vi "0_PlanVirtualStave.vi"(7 "Stave Locking Points [mm]":dbl[][](array[numeric])=[[0.0, 0.0, 0.0], [280.05, 0.0, 0.0], [574.05, 0.0, 0.0], [868.05, 0.0, 0.0], [1162.05, 0.0, 0.0]], 8 "Working height [mm]":dbl, 9 "N Modules":i32=13, 10 "Module fiducial marker":T3(ring), 11 "Tape Type":enum16{"Stereo", "Axial"}(ring)=enum."Axial") -> (0 "Module fiducials in the Stave's basis":T1(graph)=[{"Generated List of Module Coordinates"=[0.0, 280.05, 574.05, 868.05, 1162.05], "Generated List of Module Coordinates"=[0.0, 0.0, 0.0, 0.0, 0.0]}, {"Generated List of Module Coordinates"=[-7.689999999999998, 87.79, 87.79, -7.689999999999998, 90.31, 185.79000000000002, 185.79000000000002, 90.31, 188.31, 283.79, 283.79, 188.31, 286.31, 381.79, 381.79, 286.31, 384.31, 479.79, 479.79, 384.31, 482.30999999999995, 577.79, 577.79, 482.30999999999995, 580.31, 675.79, 675.79, 580.31, 678.31, 773.79, 773.79, 678.31, 776.31, 871.79, 871.79, 776.31, 874.31, 969.79, 969.79, 874.31, 972.31, 1067.79, 1067.79, 972.31, 1070.31, 1165.79, 1165.79, 1070.31, 1168.31, 1263.79, 1263.79, 1168.31], "Generated List of Module Coordinates"=[-113.212, -113.212, -16.13199999999999, -16.13199999999999, -113.212, -113.212, -16.13199999999999, -16.13199999999999, -113.212, -113.212, -16.13199999999999, -16.13199999999999, -113.212, -113.212, -16.13199999999999, -16.13199999999999, -113.212, -113.212, -16.13199999999999, -16.13199999999999, -113.212, -113.212, -16.13199999999999, -16.13199999999999, -113.212, -113.212, -16.13199999999999, -16.13199999999999, -113.212, -113.212, -16.13199999999999, -16.13199999999999, -113.212, -113.212, -16.13199999999999, -16.13199999999999, -113.212, -113.212, -16.13199999999999, -16.13199999999999, -113.212, -113.212, -16.13199999999999, -16.13199999999999, -113.212, -113.212, -16.13199999999999, -16.13199999999999, -113.212, -113.212, -16.13199999999999, -16.13199999999999]}, {"Generated List of Module Coordinates"=[40.050000000000004, 138.05, 236.05, 334.05, 432.05, 530.05, 628.05, 726.05, 824.05, 922.05, 1020.05, 1118.05, 1216.05], "Generated List of Module Coordinates"=[-64.672, -64.672, -64.672, -64.672, -64.672, -64.672, -64.672, -64.672, -64.672, -64.672, -64.672, -64.672, -64.672]}], 3 "Stave Basis: Coordinates of Fiducials on Modules":dbl[][](array[numeric])=[[-7.689999999999998, -113.212, 0.0], [87.79, -113.212, 0.0], [87.79, -16.13199999999999, 0.0], [-7.689999999999998, -16.13199999999999, 0.0], [90.31, -113.212, 0.0], [185.79000000000002, -113.212, 0.0], [185.79000000000002, -16.13199999999999, 0.0], [90.31, -16.13199999999999, 0.0], [188.31, -113.212, 0.0], [283.79, -113.212, 0.0], [283.79, -16.13199999999999, 0.0], [188.31, -16.13199999999999, 0.0], [286.31, -113.212, 0.0], [381.79, -113.212, 0.0], [381.79, -16.13199999999999, 0.0], [286.31, -16.13199999999999, 0.0], [384.31, -113.212, 0.0], [479.79, -113.212, 0.0], [479.79, -16.13199999999999, 0.0], [384.31, -16.13199999999999, 0.0], [482.30999999999995, -113.212, 0.0], [577.79, -113.212, 0.0], [577.79, -16.13199999999999, 0.0], [482.30999999999995, -16.13199999999999, 0.0], [580.31, -113.212, 0.0], [675.79, -113.212, 0.0], [675.79, -16.13199999999999, 0.0], [580.31, -16.13199999999999, 0.0], [678.31, -113.212, 0.0], [773.79, -113.212, 0.0], [773.79, -16.13199999999999, 0.0], [678.31, -16.13199999999999, 0.0], [776.31, -113.212, 0.0], [871.79, -113.212, 0.0], [871.79, -16.13199999999999, 0.0], [776.31, -16.13199999999999, 0.0], [874.31, -113.212, 0.0], [969.79, -113.212, 0.0], [969.79, -16.13199999999999, 0.0], [874.31, -16.13199999999999, 0.0], [972.31, -113.212, 0.0], [1067.79, -113.212, 0.0], [1067.79, -16.13199999999999, 0.0], [972.31, -16.13199999999999, 0.0], [1070.31, -113.212, 0.0], [1165.79, -113.212, 0.0], [1165.79, -16.13199999999999, 0.0], [1070.31, -16.13199999999999, 0.0], [1168.31, -113.212, 0.0], [1263.79, -113.212, 0.0], [1263.79, -16.13199999999999, 0.0], [1168.31, -16.13199999999999, 0.0]])   [LabVIEW 2016]
panel:
  in  "Sensor Pattern":enum16{"ATLAS07", "ATLAS12", "ATLAS17"}(ring)=enum."ATLAS12"
  in  "Stereo Angle [mrad]":dbl=40.0 format="%#_13g"
  in  "Module centre [mm]":T2
  in  "Module width [mm]":dbl=97.54
  in  "Module pitch [mm]":dbl=98.0
  # "Provided by Camera Calibration:"
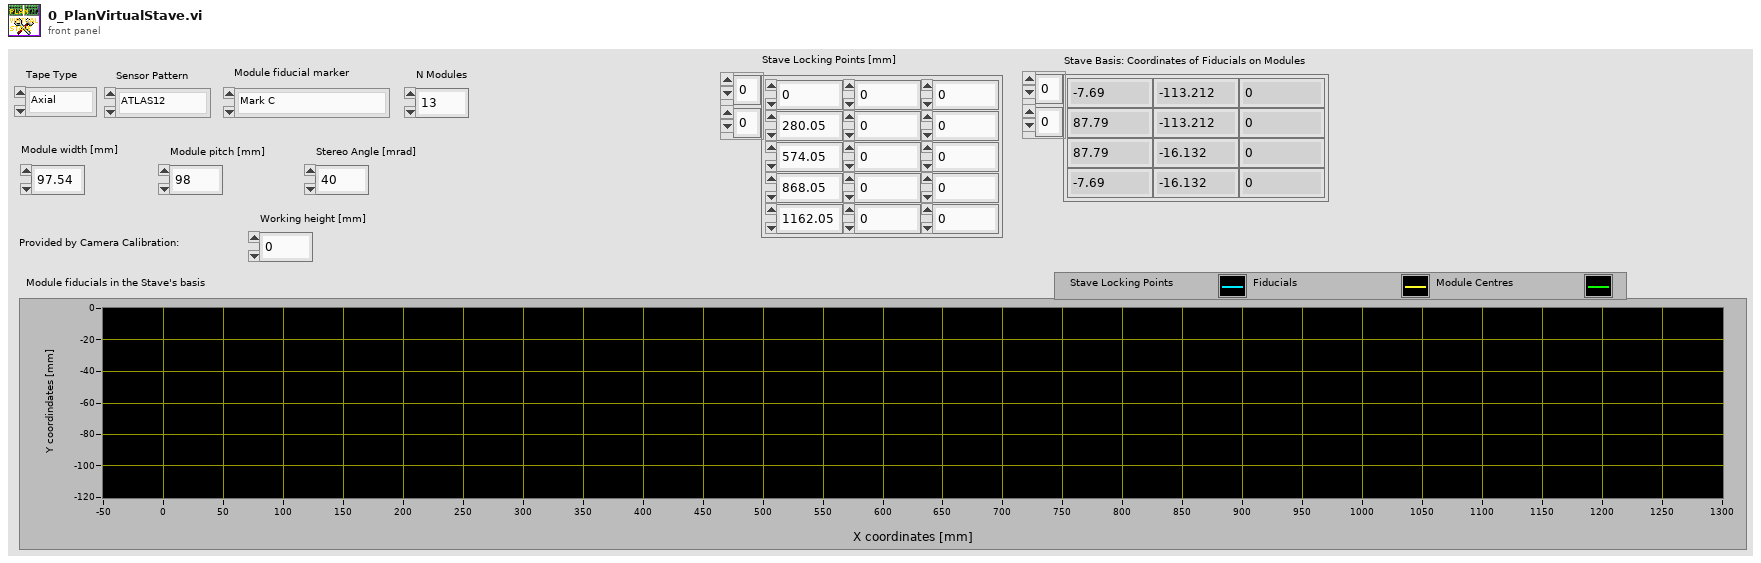
[diagram p1: front panel]
types:
  T1 = cluster{"Generated List of Module Coordinates":dbl[], "Generated List of Module Coordinates":dbl[]}[]
  T2 = cluster{"X [mm]":dbl, "Y [mm]":dbl, "Z [mm]":dbl}
  T3 = enum16{"Mark C", "Mark B", "Strip Corner", "[None]"}
  T4 = cluster{"Stave Locking Points [mm]":dbl[], "Stave Locking Points [mm]":dbl[]}
  T5 = cluster{"Generated List of Module Coordinates":dbl[], "Generated List of Module Coordinates":dbl[]}
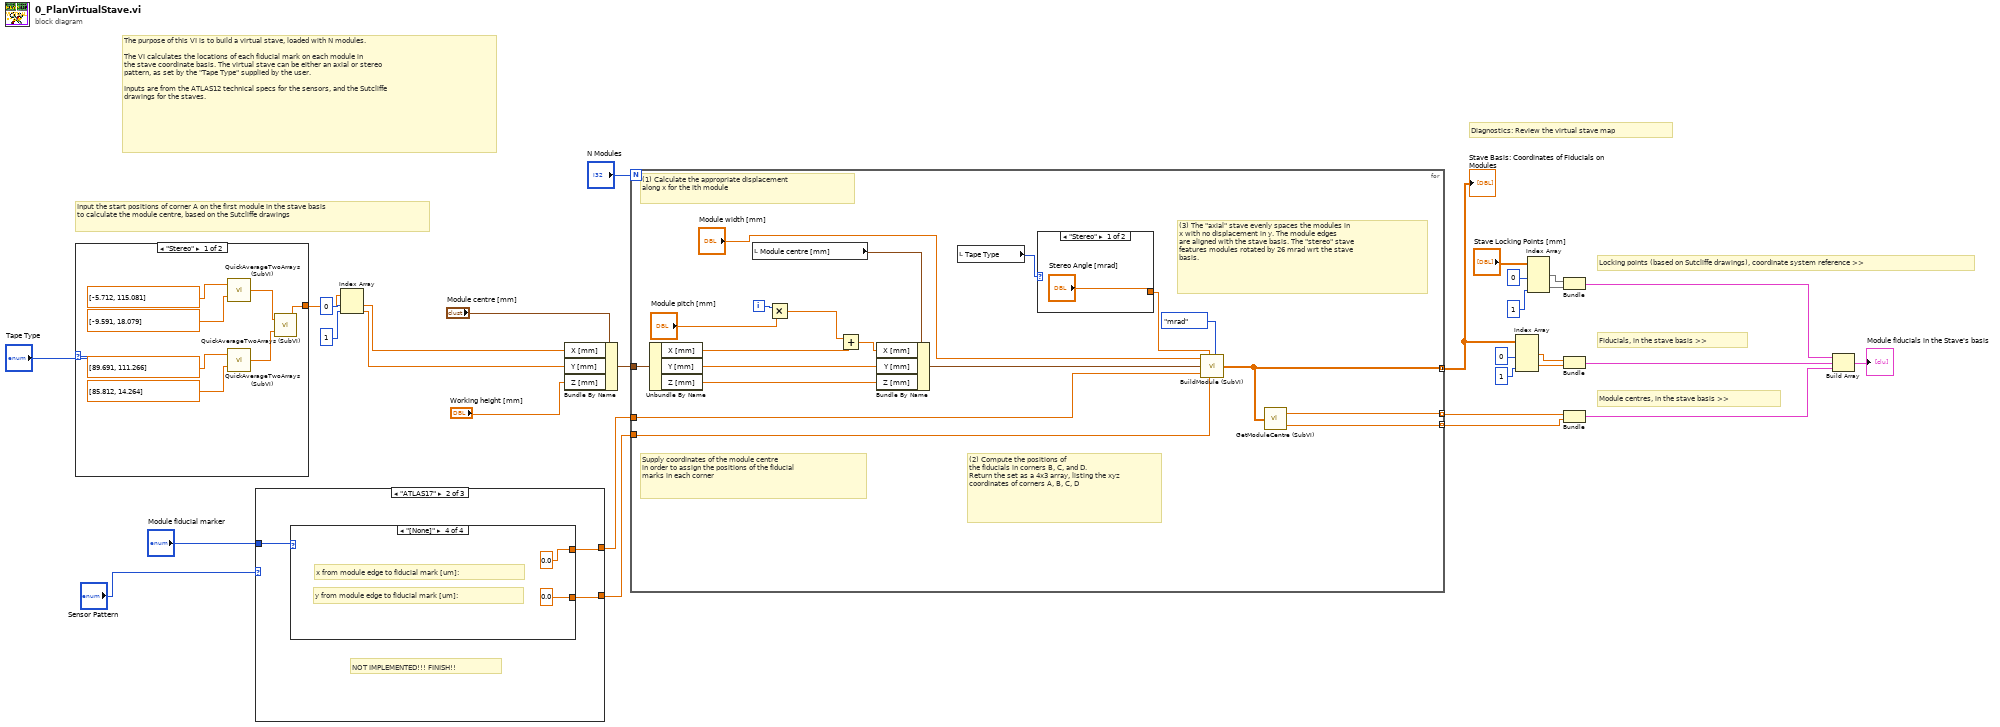
[diagram p0: block diagram]
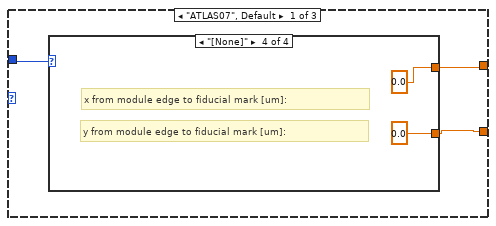
[diagram p2: hidden frame]
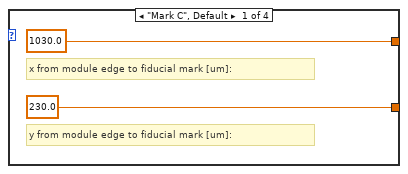
[diagram p3: hidden frame]
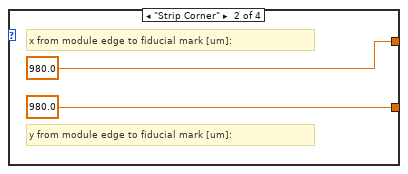
[diagram p4: hidden frame]
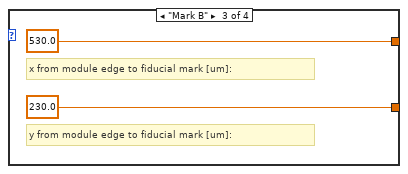
[diagram p5: hidden frame]
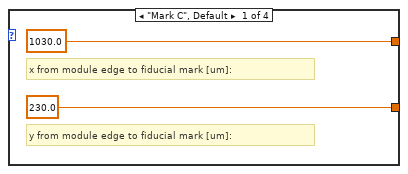
[diagram p6: hidden frame]
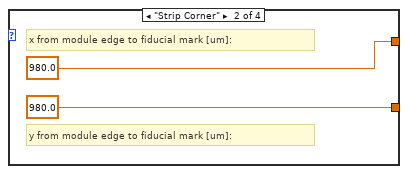
[diagram p7: hidden frame]
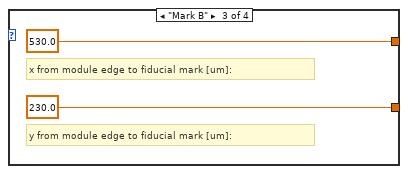
[diagram p8: hidden frame]
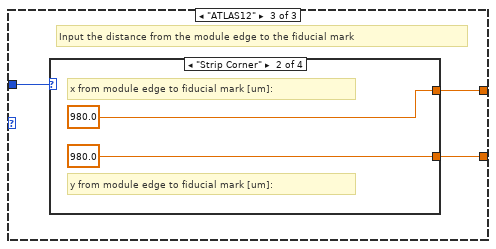
[diagram p9: hidden frame]
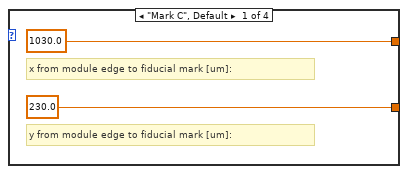
[diagram p10: hidden frame]
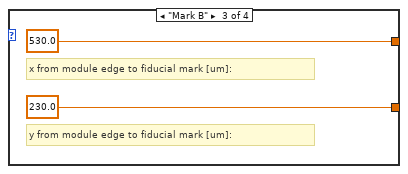
[diagram p11: hidden frame]
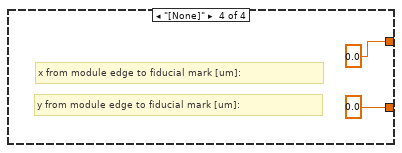
[diagram p12: hidden frame]
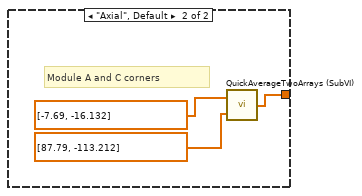
[diagram p13: hidden frame]
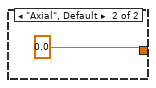
[diagram p14: hidden frame]
diagram:
  # "Locking points (based on Sutcliffe drawings), coordinate system reference >>"
  # "Module centres, in the stave basis >>"
  # "Fiducials, in the stave basis >>"
  # "Diagnostics: Review the virtual stave map"
  # "Input the start positions of corner A on the first module in the stave basis\nto calculate the module centre, based on the Sutcliffe drawings"
  # "The purpose of this VI is to build a virtual stave, loaded with N modules.\n\nThe VI calculates the locations of each fiducial mark on each module in \nthe stave coordinate basis. The virtual stave can be either an axial or stereo \npattern, as set by the \"Tape Type\" supplied by the user.\n\nInputs are from the ATLAS12 technical specs for the sensors, and the Sutcliffe\ndrawings for the staves."
  n1 = case shown="\"Stereo\"" "Tape Type" {
    tunnel: [w31 w38] -> w4
    frame "Stereo" {
      n2 = call "QuickAverageTwoArrays (SubVI).vi"("B"=dbl[] [-9.591, 18.079], "A"=dbl[] [-5.712, 115.081]) -> ("Average of A and B"=w36:dbl[])
      n3 = call "QuickAverageTwoArrays (SubVI).vi"("B"=dbl[] [85.812, 14.264], "A"=dbl[] [89.691, 111.266]) -> ("Average of A and B"=w37:dbl[])
      n4 = call "QuickAverageTwoArrays (SubVI).vi"("B"=w37, "A"=w36) -> ("Average of A and B"=w31:dbl[])
    }
    frame "Axial", Default {
      # "Module A and C corners"
      n5 = call "QuickAverageTwoArrays (SubVI).vi"("B"=dbl[] [87.79, -113.212], "A"=dbl[] [-7.69, -16.132]) -> ("Average of A and B"=w38:dbl[])
    }
  }
  n6 = case shown="\"ATLAS17\"" "Sensor Pattern" {
    tunnel: "Module fiducial marker" -> [w43 w54 w65]
    tunnel: [w42 w53 w64] -> w29
    tunnel: [w41 w52 w63] -> w28
    frame "ATLAS07", Default {
      n7 = case shown="\"[None]\"" w43 {
        tunnel: [1030.0 980.0 530.0 0.0] -> w42
        tunnel: [230.0 980.0 230.0 0.0] -> w41
        frame "Mark C", Default {
          # "y from module edge to fiducial mark [um]:"
          # "x from module edge to fiducial mark [um]:"
        }
        frame "Strip Corner" {
          # "y from module edge to fiducial mark [um]:"
          # "x from module edge to fiducial mark [um]:"
        }
        frame "Mark B" {
          # "y from module edge to fiducial mark [um]:"
          # "x from module edge to fiducial mark [um]:"
        }
        frame "[None]" {
          # "y from module edge to fiducial mark [um]:"
          # "x from module edge to fiducial mark [um]:"
        }
      }
    }
    frame "ATLAS17" {
      # "NOT IMPLEMENTED!!! FINISH!!"
      n8 = case shown="\"[None]\"" w54 {
        tunnel: [1030.0 980.0 530.0 0.0] -> w53
        tunnel: [230.0 980.0 230.0 0.0] -> w52
        frame "Mark C", Default {
          # "y from module edge to fiducial mark [um]:"
          # "x from module edge to fiducial mark [um]:"
        }
        frame "Strip Corner" {
          # "y from module edge to fiducial mark [um]:"
          # "x from module edge to fiducial mark [um]:"
        }
        frame "Mark B" {
          # "y from module edge to fiducial mark [um]:"
          # "x from module edge to fiducial mark [um]:"
        }
        frame "[None]" {
          # "y from module edge to fiducial mark [um]:"
          # "x from module edge to fiducial mark [um]:"
        }
      }
    }
    frame "ATLAS12" {
      # "Input the distance from the module edge to the fiducial mark"
      n9 = case shown="\"Strip Corner\"" w65 {
        tunnel: [1030.0 980.0 530.0 0.0] -> w64
        tunnel: [230.0 980.0 230.0 0.0] -> w63
        frame "Mark C", Default {
          # "y from module edge to fiducial mark [um]:"
          # "x from module edge to fiducial mark [um]:"
        }
        frame "Strip Corner" {
          # "y from module edge to fiducial mark [um]:"
          # "x from module edge to fiducial mark [um]:"
        }
        frame "Mark B" {
          # "y from module edge to fiducial mark [um]:"
          # "x from module edge to fiducial mark [um]:"
        }
        frame "[None]" {
          # "y from module edge to fiducial mark [um]:"
          # "x from module edge to fiducial mark [um]:"
        }
      }
    }
  }
  n10 = Index Array(array=w4, index #1=0 ("index"), index #2=1 ("index")) -> (element #1=w8:dbl, element #2=w6:dbl)
  n11 = Bundle By Name(cluster="Module centre [mm]", "X [mm]"=w8, "Y [mm]"=w6, "Z [mm]"="Working height [mm]") -> (w23:T2)
  n12 = for {
    N: "N Modules" -> [_]
    tunnel: w29 -> [w82]
    tunnel: w28 -> [w92]
    tunnel: w23 -> [w81]
    tunnel: [w74] -> w17 mode=concatenating
    tunnel: [w80] -> w14 mode=indexing
    tunnel: [w79] -> w3 mode=indexing
    i -> [w91]
    # "(3) The \"axial\" stave evenly spaces the modules in \nx with no displacement in y. The module edges \nare aligned with the stave basis. The \"stereo\" stave \nfeatures modules rotated by 26 mrad wrt the stave\nbasis."
    # "(2) Compute the positions of \nthe fiducials in corners B, C, and D. \nReturn the set as a 4x3 array, listing the xyz coordinates of corners A, B, C, D"
    # "(1) Calculate the appropriate displacement \nalong x for the ith module"
    # "Supply coordinates of the module centre \nin order to assign the positions of the fiducial \nmarks in each corner"
    n13 = Unbundle By Name(w81) -> ("X [mm]"=w90:dbl, "Y [mm]"=w88:dbl, "Z [mm]"=w86:dbl)
    n14 = local read "Module centre [mm]"() -> (w84:T2)
    n15 = Multiply(x=w91, y="Module pitch [mm]") -> (x*y=w89:dbl)
    n16 = Add(x=w89, y=w90) -> (x+y=w87:dbl)
    n17 = Bundle By Name(cluster=w84, "X [mm]"=w87, "Y [mm]"=w88, "Z [mm]"=w86) -> (w85:T2)
    n18 = local read "Tape Type"() -> (w76:enum16{"Stereo", "Axial"})
    n19 = case shown="\"Stereo\"" w76 {
      tunnel: ["Stereo Angle [mrad]" 0.0 ("Angle")] -> w75
      frame "Stereo" {
      }
      frame "Axial", Default {
      }
    }
    n20 = call "BuildModule (SubVI).vi"("Module side length [mm]"="Module width [mm]", "Angle"=w75, "Centre [mm]"=w85, "x to fiducial [um]"=w82, "y to fiducial [um]"=w92, "Units"=enum16{"mrad", "Radians", "Degrees"}."mrad") -> ("Generated List of Module Coordinates"=w74:dbl[][])  [unwired: 3 in]
    n21 = call "GetModuleCentre (SubVI).vi"("4x3 Array of Fiducial Coordinates"=w74) -> ("x, centre"=w80:dbl, "y, centre"=w79:dbl)
  }
  "Stave Basis: Coordinates of Fiducials on Modules" <- w17
  n22 = Index Array(array=w17, index (col) #1=0 ("disabled index (col)"), index (col) #2=1 ("index (col)")) -> (element #1=w27:dbl[], element #2=w26:dbl[])  [unwired: 2 in]
  n23 = Index Array(array="Stave Locking Points [mm]", index (col) #1=0 ("disabled index (col)"), index (col) #2=1 ("disabled index (col)")) -> (element #1=w19:dbl[], element #2=w18:dbl[])  [unwired: 2 in]
  n24 = Bundle("Stave Locking Points [mm]"=w19, "Stave Locking Points [mm]"=w18) -> (w11:T4)  [unwired: 1 in]
  n25 = Bundle("Generated List of Module Coordinates"=w27, "Generated List of Module Coordinates"=w26) -> (w13:T5)  [unwired: 1 in]
  n26 = Bundle(w14, w3) -> (w12:cluster{dbl[], dbl[]})  [unwired: 1 in]
  n27 = Build Array(w11, w13, w12) -> (→"Module fiducials in the Stave's basis":T1)
